vi "SaveBlock.vi"(6 "registry":T12, 8 "error in (no error)":errorcluster, 9 "data flow":T16, 10 "data event config":T1, 11 "data event":T4) -> (0 "error out":errorcluster, 2 "data event config out":T1, 3 "data event out":T4)   [LabVIEW 2017, in "EmsaDataEventCreator.lvlib"]
uses:
  <vilib>/addons/InsightCM/Devices/Shared/Emsa/EmsaDataEventCreator/EmsaDataEventCreator.lvlib
  <vilib>/addons/InsightCM/Devices/Shared/Emsa/EmsaDataEventCreator/controls/DataEventConfig.ctl
  <vilib>/addons/PointValueMap/controls/PointMap.ctl
  <vilib>/addons/InsightCM/Devices/Shared/Emsa/EmsaDataEventCreator/controls/SweepParams.ctl
  <vilib>/addons/InsightCM/Devices/Shared/Common/DataFlow/controls/Data.ctl
  <vilib>/addons/InsightCM/Utilities/DataAccessors/controls/wfmSGL_DVR.ctl
  <vilib>/addons/InsightCM/Devices/Shared/Common/DataFlow/controls/Type.ctl
  <vilib>/addons/InsightCM/Devices/Shared/Emsa/EmsaDataEventCreator/controls/Registry.ctl
  <vilib>/addons/InsightCM/Devices/Shared/Emsa/EmsaDataEventCreator/controls/Registry_Sweep.ctl
  <vilib>/addons/InsightCM/Devices/Shared/Common/DataEvent/controls/DataSetType.ctl
  <vilib>/addons/InsightCM/MessageBus/Base/controls/KeyValuePair.ctl
  <vilib>/addons/InsightCM/Devices/Shared/Common/DataEventCreator/controls/Registry_Trend.ctl
  <vilib>/addons/InsightCM/Devices/Shared/Common/DataEvent/controls/Event.ctl
  <vilib>/addons/InsightCM/MessageBus/Base/controls/DataEvent.ctl
  <vilib>/addons/InsightCM/Devices/Shared/Common/DataEvent/controls/DataSet.ctl
  <vilib>/addons/InsightCM/MessageBus/Base/controls/DataSetMetadata.ctl
  <vilib>/addons/InsightCM/MessageBus/Base/controls/TrendPoint.ctl
  <vilib>/addons/InsightCM/MessageBus/Base/controls/TrendAlarmUpdate.ctl
  <vilib>/addons/InsightCM/MessageBus/Base/controls/TrendAlarmTransition.ctl
  <vilib>/addons/InsightCM/Utilities/PropertyHelpers/PropertyHelpers.lvlib
  <vilib>/addons/InsightCM/Devices/Shared/Common/DataEventCreator/DataEventCreator.lvlib
  <vilib>/addons/InsightCM/Devices/Shared/Emsa/EmsaAcquisition/EmsaAcquisition.lvlib
  <vilib>/addons/PointValueMap/PointValueMap.lvlib
  <vilib>/addons/InsightCM/Devices/Shared/Common/DataFlow/DataFlow.lvlib
  <vilib>/addons/InsightCM/Devices/Shared/Common/DataEvent/DataEvent.lvlib
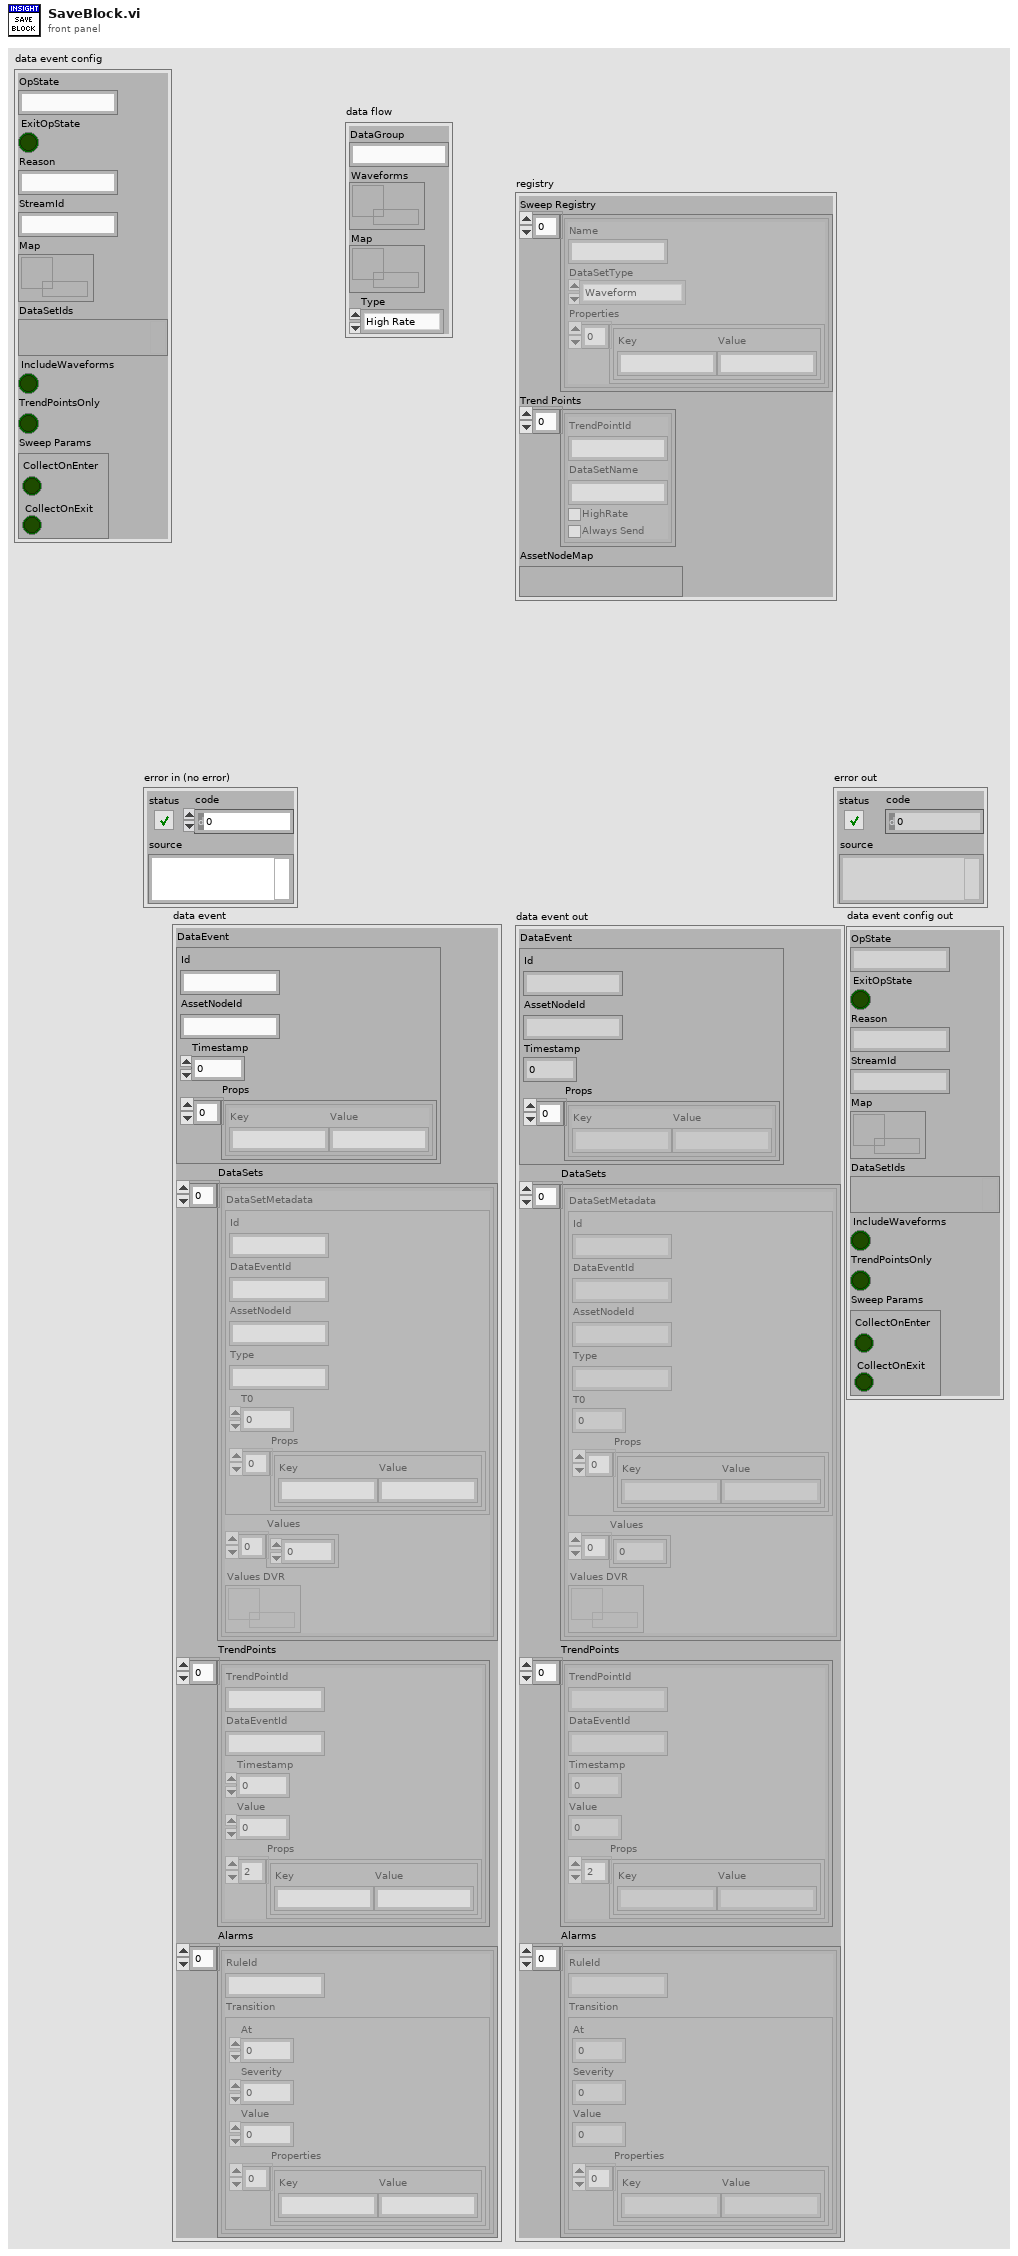
[diagram p1: front panel]
types:
  T1 = typedef "EmsaDataEventCreator.lvlib/DataEventConfig.ctl" = cluster{"OpState":string, "ExitOpState":bool, "Reason":string, "StreamId":string, "Map":T2, "DataSetIds":variant, "IncludeWaveforms":bool, "TrendPointsOnly":bool, "Sweep Params":T3}
  T2 = typedef "PointValueMap.lvlib/PointMap.ctl" = refnum<data-value>
  T3 = typedef "EmsaDataEventCreator.lvlib/SweepParams.ctl" = cluster{"CollectOnEnter":bool, "CollectOnExit":bool}
  T4 = typedef "DataEvent.lvlib/Event.ctl" = cluster{"DataEvent":T5, "DataSets":T7[], "TrendPoints":T9[], "Alarms":T10[]}
  T5 = typedef "DataEvent.ctl" = cluster{"Id":string, "AssetNodeId":string, "Timestamp":i64, "Props":T6[]}
  T6 = typedef "KeyValuePair.ctl" = cluster{"Key":string, "Value":string}
  T7 = typedef "DataEvent.lvlib/DataSet.ctl" = cluster{"DataSetMetadata":T8, "Values":sgl[], "Values DVR":refnum<data-value>}
  T8 = typedef "DataSetMetadata.ctl" = cluster{"Id":string, "DataEventId":string, "AssetNodeId":string, "Type":string, "T0":i64, "Props":T6[]}
  T9 = typedef "TrendPoint.ctl" = cluster{"TrendPointId":string, "DataEventId":string, "Timestamp":i64, "Value":dbl, "Props":T6[]}
  T10 = typedef "TrendAlarmUpdate.ctl" = cluster{"RuleId":string, "Transition":T11}
  T11 = typedef "TrendAlarmTransition.ctl" = cluster{"At":i64, "Severity":i32, "Value":dbl, "Properties":T6[]}
  T12 = typedef "EmsaDataEventCreator.lvlib/Registry.ctl" = cluster{"Sweep Registry":T13[], "Trend Points":T15[], "AssetNodeMap":variant}
  T13 = typedef "EmsaDataEventCreator.lvlib/Registry_Sweep.ctl" = cluster{"Name":string, "DataSetType":T14, "Properties":T6[]}
  T14 = typedef "DataEvent.lvlib/DataSetType.ctl" = enum16{"Waveform", "SpeedProfile", "ThermalImage", "EmsaSweep"}
  T15 = typedef "DataEventCreator.lvlib/Registry_Trend.ctl" = cluster{"TrendPointId":string, "DataSetName":string, "HighRate":bool, "Always Send":bool}
  T16 = typedef "DataFlow.lvlib/Data.ctl" = cluster{"DataGroup":string, "Waveforms":T17, "Map":T2, "Type":T18}
  T17 = typedef "wfmSGL_DVR.ctl" = refnum<data-value>
  T18 = typedef "DataFlow.lvlib/Type.ctl" = enum16{"High Rate", "Low Rate", "Burst Mode"}
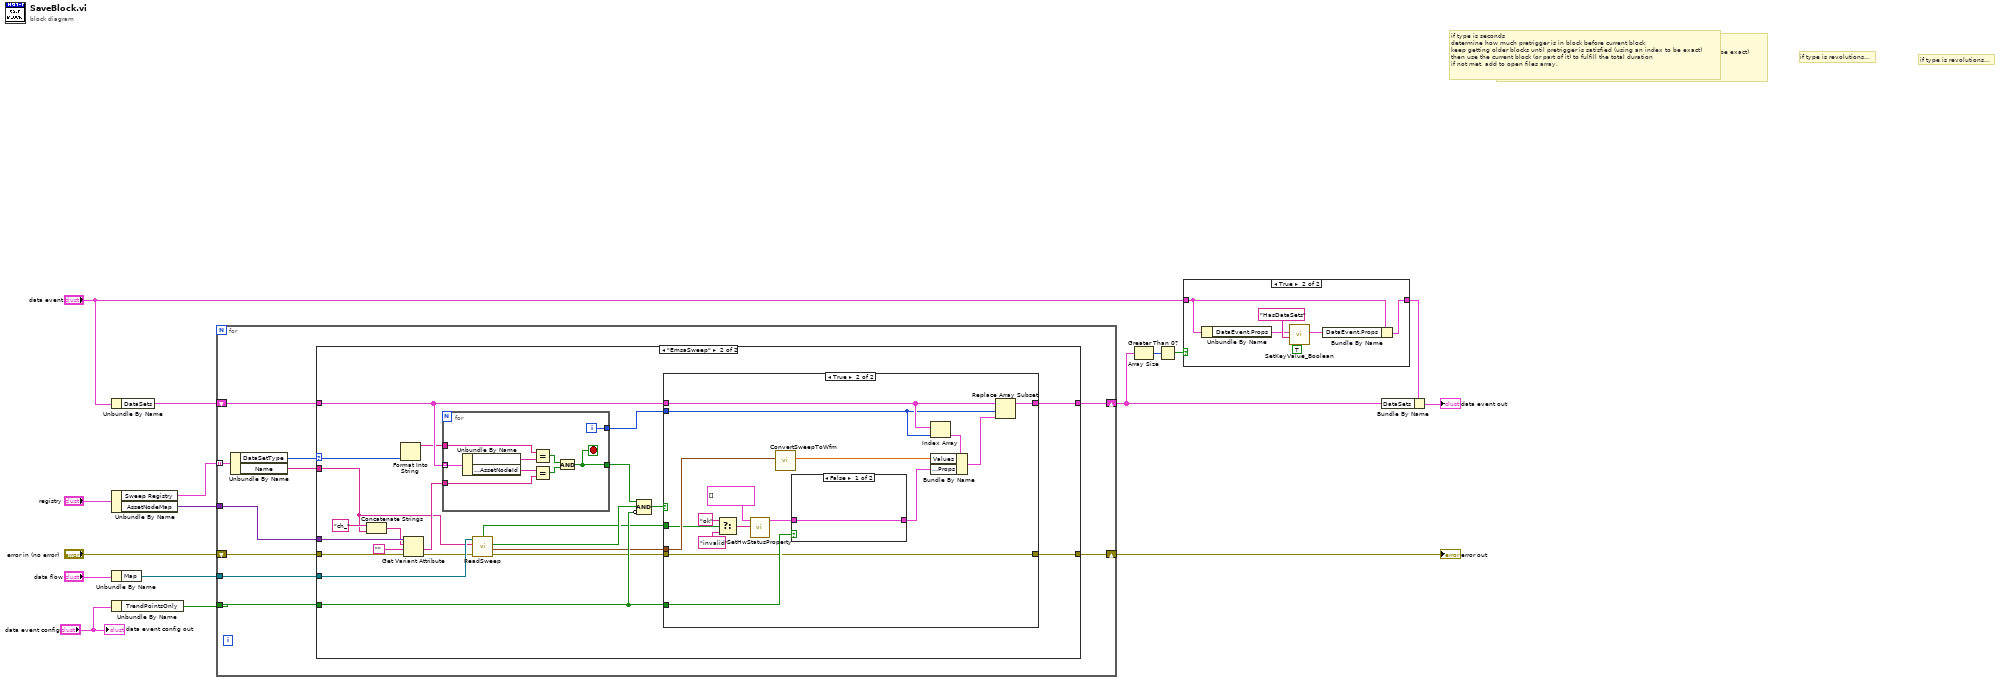
[diagram p0: block diagram]
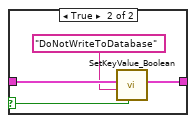
[diagram p5: hidden frame]
diagram:
  # "if type is revolutions..."
  # "if type is seconds\ndetermine how much pretrigger is in block before current block\nkeep getting older blocks until pretrigger is satisfied (using an index to be exact)\nthen use the current block (or part of it) to fulfill the total duration\nif not met, add to open files array."
  # "if type is revolutions..."
  # "if type is seconds\ndetermine how much pretrigger is in block before current block\nkeep getting older blocks until pretrigger is satisfied (using an index to be exact)\nthen use the current block (or part of it) to fulfill the total duration\nif not met, add to open files array."
  n1 = Unbundle By Name("data event") -> ("DataSets"=w10:T7[])
  n2 = Unbundle By Name("registry") -> ("Sweep Registry"=w9:T13[], "AssetNodeMap"=w11:variant)
  n3 = Unbundle By Name("data flow") -> ("Map"=w14:T2)
  n4 = Unbundle By Name("data event config") -> ("TrendPointsOnly"=w15:bool)
  n5 = for {
    tunnel: w15 -> [w20]
    tunnel: w14 -> [w26]
    tunnel: w11 -> [w22]
    tunnel: w9 -> [w25] mode=indexing
    shift-right: [w19] -> w7
    shift-left: "error in (no error)" -> [w23]
    shift-right: [w17] -> w1
    shift-left: w10 -> [w24]
    n6 = Unbundle By Name(w25) -> ("DataSetType"=w18:T14, "Name"=w21:string)
    n7 = case shown="\"EmsaSweep\"" w18 {
      selector: w18 -> [_ w38]
      tunnel: w26 -> [_ w37]
      tunnel: [w28 w50] -> w17
      tunnel: w24 -> [w28 w49]
      tunnel: w23 -> [w27 w48]
      tunnel: w22 -> [_ w47]
      tunnel: w21 -> [_ w30]
      tunnel: w20 -> [_ w43]
      tunnel: [w27 w39] -> w19
      frame Default {
      }
      frame "EmsaSweep" {
        n8 = Concatenate Strings("ch_" ("string"), w30) -> (w29:string)
        n9 = Format Into String(w38) -> (resulting string=w44:string)  [unwired: 3 in, 1 out]
        n10 = Get Variant Attribute(Variant=w47, name=w29, default value (empty Variant)="", error in=w48) -> (value=w45:string, error out=w34:errorcluster)  [unwired: 2 out]
        n11 = for {
          tunnel: w49 -> [w59] mode=indexing
          tunnel: w45 -> [w55]
          tunnel: w44 -> [w57]
          tunnel: [w52] -> w42
          tunnel: [w51] -> w40
          i -> [w51]
          stop <- w52 stop-if-true
          n12 = Unbundle By Name(w59) -> ("DataSetMetadata.Type"=w58:string, "DataSetMetadata.AssetNodeId"=w56:string)
          n13 = Equal?(x=w57, y=w58) -> (x = y?=w54:bool)
          n14 = Equal?(x=w56, y=w55) -> (x = y?=w53:bool)
          n15 = And(x=w54, y=w53) -> (x .and. y?=w52:bool)
        }
        n16 = call <vilib>:"ReadSweep.vi"("error in (no error)"=w34, "channel"=w30, "map"=w37) -> ("error out"=w33:errorcluster, "sweep"=w35:cluster{"frequency":dbl, "amplitude":dbl}[], "found"=w36:bool, "valid"=w32:bool)  [unwired: 3 in, 2 out]
        n17 = Compound Arithmetic op=AND(w42, w36, invert w43) -> (w41:bool)
        n18 = case shown="True" w41 {
          tunnel: w49 -> [w61 w64]
          tunnel: [w61 w73] -> w50
          tunnel: w43 -> [_ w77]
          tunnel: w35 -> [_ w69]
          tunnel: w33 -> [w60 w70]
          tunnel: w40 -> [_ w63]
          tunnel: [w60 w70] -> w39
          tunnel: w32 -> [_ w68]
          frame False {
          }
          frame True {
            n19 = Select(t="ok" ("hw status"), s=w68, f="invalid") -> (s? t:f=w66:string)
            n20 = call <vilib>:"SetHwStatusProperty.vi"("hw status"=w66, "props in"=T6[] [] ("key value pairs")) -> ("props out"=w74:T6[])  [unwired: 9 in]
            n21 = call <vilib>:"ConvertSweepToWfm.vi"("sweep"=w69) -> ("array"=w76:sgl[])  [unwired: 10 in]
            n22 = case shown="False" w77 {
              selector: w77 -> [_ w79]
              tunnel: w74 -> [w78 w82]
              tunnel: [w78 w81] -> w72
              frame False {
              }
              frame True {
                n23 = call <vilib>:"SetKeyValue_Boolean.vi"("value"=w79, "key"="DoNotWriteToDatabase", "key value pairs"=w82) -> ("key value pairs out"=w81:T6[])  [unwired: 8 in]
              }
            }
            n24 = Index Array(array=w64, index=w63) -> (element=w62:T7)
            n25 = Bundle By Name(cluster=w62, "Values"=w76, "DataSetMetadata.Props"=w72) -> (w71:T7)
            n26 = Replace Array Subset(array=w64, new element=w71, index=w63) -> (w73:T7[])
          }
        }
      }
    }
  }
  "error out" <- w7
  n27 = Array Size(array=w1) -> (size(s)=w5:i32)
  n28 = Greater Than 0?(x=w5) -> (x > 0?=w4:bool)
  n29 = case shown="True" w4 {
    tunnel: [w83 w84] -> w2
    tunnel: "data event" -> [w83 w86]
    frame False {
    }
    frame True {
      n30 = Unbundle By Name(w86) -> ("DataEvent.Props"=w87:T6[])
      n31 = call <vilib>:"SetKeyValue_Boolean.vi"("value"=TRUE, "key"="HasDataSets", "key value pairs"=w87) -> ("key value pairs out"=w85:T6[])  [unwired: 8 in]
      n32 = Bundle By Name(cluster=w86, "DataEvent.Props"=w85) -> (w84:T4)
    }
  }
  n33 = Bundle By Name(cluster=w2, "DataSets"=w1) -> (→"data event out":T4)
  "data event config out" <- "data event config"
